vi "Rename Document.vi"() -> ()   [LabVIEW 2019]
uses:
  _SubVI/Cluster.ctl
  <userlib>/IoT Devices/_subVIs/HTTPComm.ctl
panel:
  out "Comm":T1
  in  "cancel":bool
  out "error out":errorcluster
  in  "error in":errorcluster
  in  "Device In":T2
  out "Device Out":T2
  in  "OK Button":bool
  in  "List of files":u16(ring) items=["hainahola", "pepsi", "Okay sure", "milan", "changed doc", "renamed name", "ds", "latest doc", "milan", "latest doc", "milan", "something", "qq", "HELLO MILAN boss", "very cool", "HELLO MILAN", "new", "OnShape_Placemat_Glasses Challenge.pdf", "Untitled document", "FeatureStudio Test"]
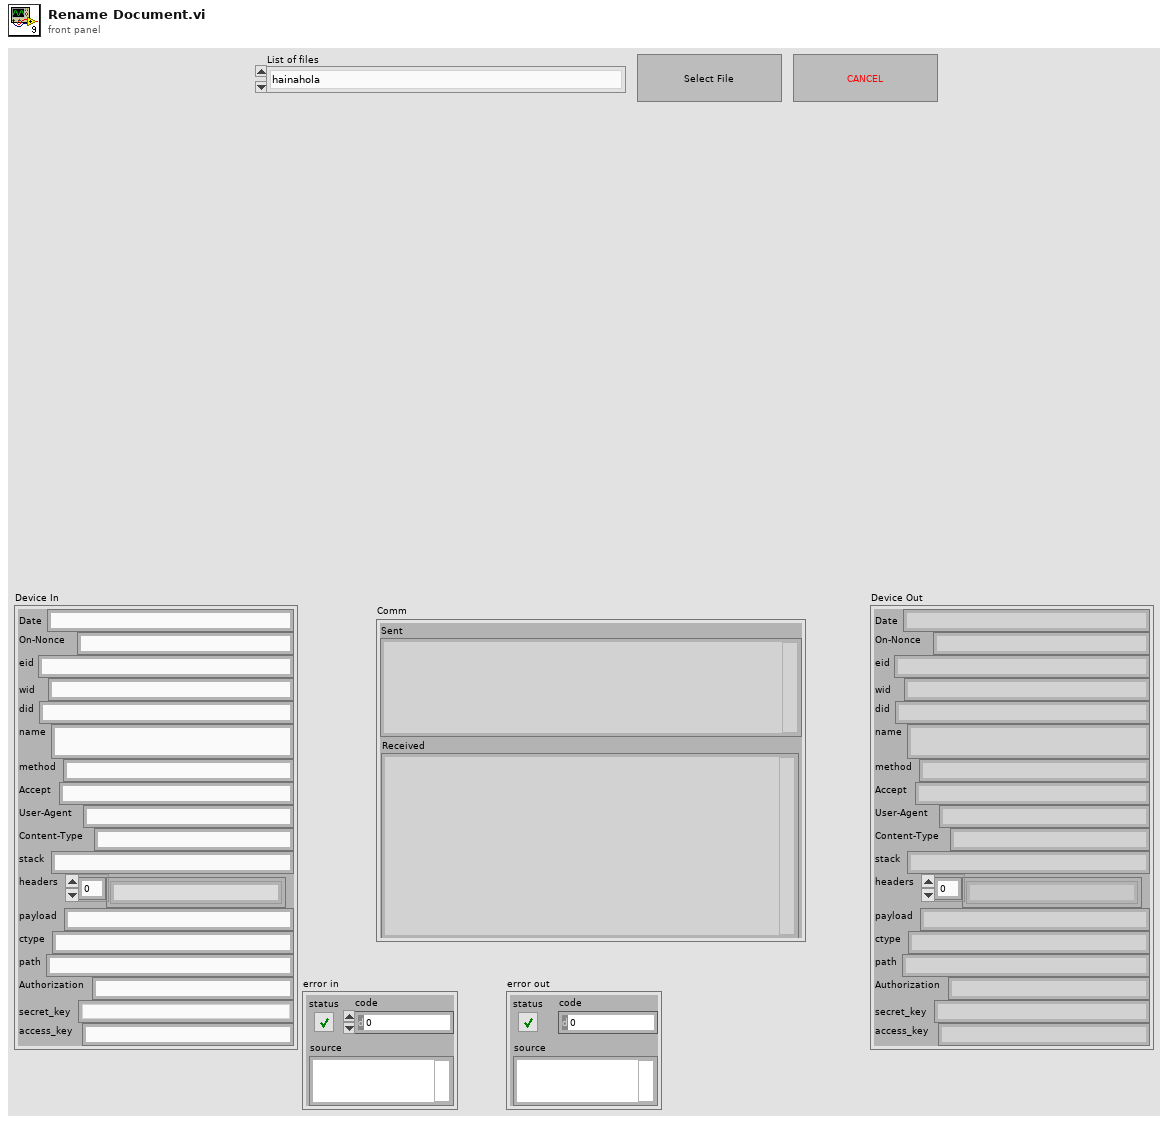
[diagram p1: front panel]
types:
  T1 = typedef "HTTPComm.ctl" = cluster{"url":string, "sent headers":string, "sent body":string, "headers":string, "body":string, "Sent":string, "Received":string}
  T2 = typedef "Cluster.ctl" = cluster{"Date":string, "On-Nonce":string, "eid":string, "wid":string, "did":string, "name":string, "method":string, "Accept":string, "User-Agent":string, "Content-Type":string, "stack":string, "headers":string[], "payload":string, "ctype":string, "path":string, "Authorization":string, "secret_key":string, "access_key":string}
  T3 = enum32{"Invalid", "Standard", "Closed", "Hidden", "Minimized", "Maximized"}
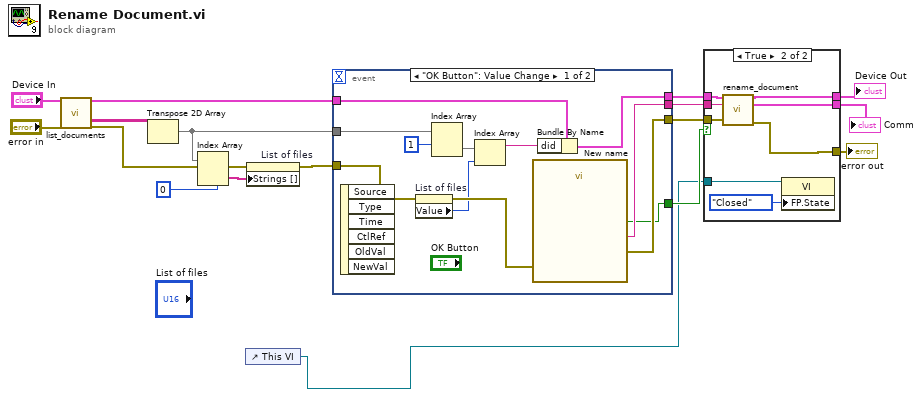
[diagram p0: block diagram]
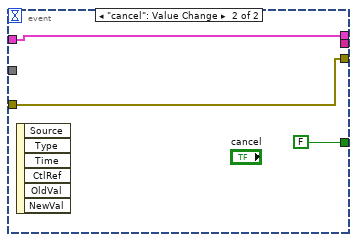
[diagram p3: hidden frame]
diagram:
  n1 = call "list_documents.vi"("Device In"="Device In", "error in"="error in") -> ("Device Out"=w17:T2, "Document list"=w16:string[][], "error out"=w13:errorcluster)  [unwired: 14 in, 1 out]
  n2 = Transpose 2D Array(2D array=w16) -> (transposed array=w11:string[][])
  n3 = Index Array(array=w11, index (row)=0) -> (element=w14:string[])  [unwired: 1 in]
  n4 = control-ref of="This VI"() -> (w1:refnum<vi>)
  n5 = property on="List of files" class="Ring (strict)"(error in=w13, "Strings []"=w14) -> (error out=w12:errorcluster)  [unwired: 1 in, 1 out]
  n6 = event shown="[0] \"OK Button\": Value Change" {
    selector: _ -> [_ _]
    dyn-events: _ -> [_ _]
    timeout: _ -> [_ _]
    tunnel: w17 -> [w29 w32]
    tunnel: w12 -> [w25 w31]
    tunnel: w11 -> [w22 _]
    tunnel: [w21 w32] -> w8
    tunnel: [w20 _] -> w7
    tunnel: [w19 w31] -> w6
    tunnel: [w18 FALSE] -> w2
    event "OK Button": Value Change {
      n7 = event-data() -> ()  [unwired: 1 in, 6 out]
      n8 = property on="List of files" class="Ring (strict)"(error in=w25) -> (error out=w24:errorcluster, "Value"=w23:u16)  [unwired: 1 in, 1 out]
      n9 = Index Array(array=w22, index (row)=1) -> (element=w28:string[])  [unwired: 1 in]
      n10 = Index Array(array=w28, index=w23) -> (element=w26:string)
      n11 = call "New name"("error in (no error)"=w24) -> ("New name"=w20:string, "Change"=w18:bool, "error out"=w19:errorcluster)  [unwired: 16 in]
      n12 = Bundle By Name(cluster=w29, "did"=w26) -> (w21:T2)
    }
    event "cancel": Value Change {
      n13 = event-data() -> ()  [unwired: 1 in, 6 out]
    }
  }
  n14 = case shown="True" w2 {
    tunnel: w8 -> [w34 w42]
    tunnel: w7 -> [_ w41]
    tunnel: w6 -> [w33 w40]
    tunnel: [w34 w39] -> w5
    tunnel: [w33 w38] -> w4
    tunnel: [_ w37] -> w3
    tunnel: w1 -> [_ w35]
    frame False {
    }
    frame True {
      n15 = call "rename_document.vi"("Device In"=w42, "New Name"=w41, "error in"=w40) -> ("Device Out"=w39:T2, "Comm"=w37:T1, "error out"=w38:errorcluster)  [unwired: 10 in]
      n16 = property class="VI"(reference=w35, "FP.State"=T3."Closed" ("Front Panel Window:State")) -> ()  [unwired: 1 in, 2 out]
    }
  }
  "Device Out" <- w5
  "error out" <- w4
  "Comm" <- w3
